vi "GetName.vi"(8 "error in (no error)":errorcluster, 11 "FakeTestSuite in":refnum<class "FakeTestSuite.lvclass">) -> (0 "error out":errorcluster, 2 "Name":string, 3 "FakeTestSuite out":refnum<class "FakeTestSuite.lvclass">)   [LabVIEW 2019, in "ResultTreeListenerTest.lvlib" / "Support.lvlib" / "FakeTestSuite.lvclass"]
doc: "Returns the name."
uses:
  FakeTestSuite.lvclass
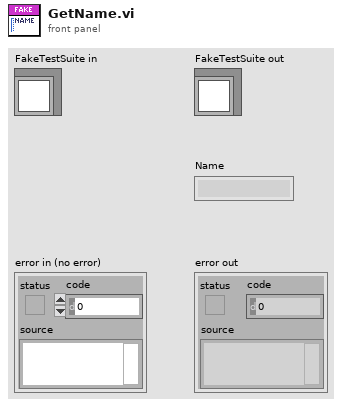
[diagram p1: front panel]
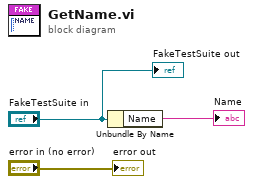
[diagram p0: block diagram]
diagram:
  n1 = Unbundle By Name("FakeTestSuite in") -> ("Name"=→"Name":string)
  "error out" <- "error in (no error)"
  "FakeTestSuite out" <- "FakeTestSuite in"
